vi "Set Channel States and Connections.vi"(8 "error in (no error)":errorcluster, 10 "Routing Channel States":T1, 11 "Channel Ref in":T4 format="%.0x") -> (0 "error out":errorcluster, 3 "Channel Ref out":T4=18446744073709551615 format="%.0x")   [LabVIEW 2017, in "Switch Scripting.lvlib"]
uses:
  Switch Scripting.lvlib
  <vilib>/NI Veristand/Custom Device API/Custom Device Item Ref.ctl
  Channel States.ctl
  Routing State.ctl
  Connection.ctl
  NationalInstruments.VeriStand.SystemDefinitionAPI
  <vilib>/NI VeriStand/Custom Device API/Custom Device API.lvlib
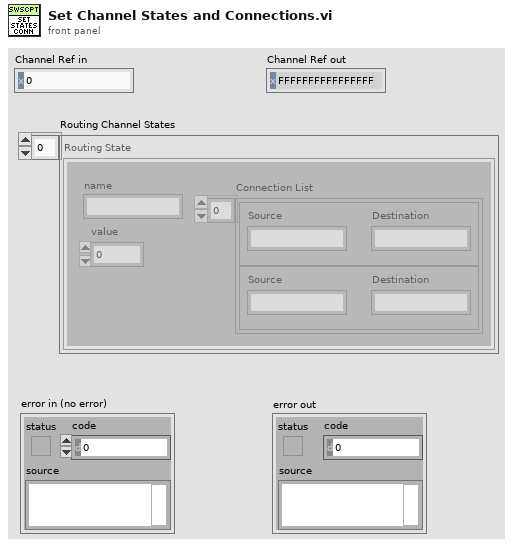
[diagram p1: front panel]
types:
  T1 = typedef "Switch Scripting.lvlib/Channel States.ctl" = T2[]
  T2 = typedef "Switch Scripting.lvlib/Routing State.ctl" = cluster{"name":string, "value":i32, "Connection List":T3[]}
  T3 = typedef "Switch Scripting.lvlib/Connection.ctl" = cluster{"Source":string, "Destination":string}
  T4 = typedef "Custom Device API.lvlib/Custom Device Item Ref.ctl" = u64
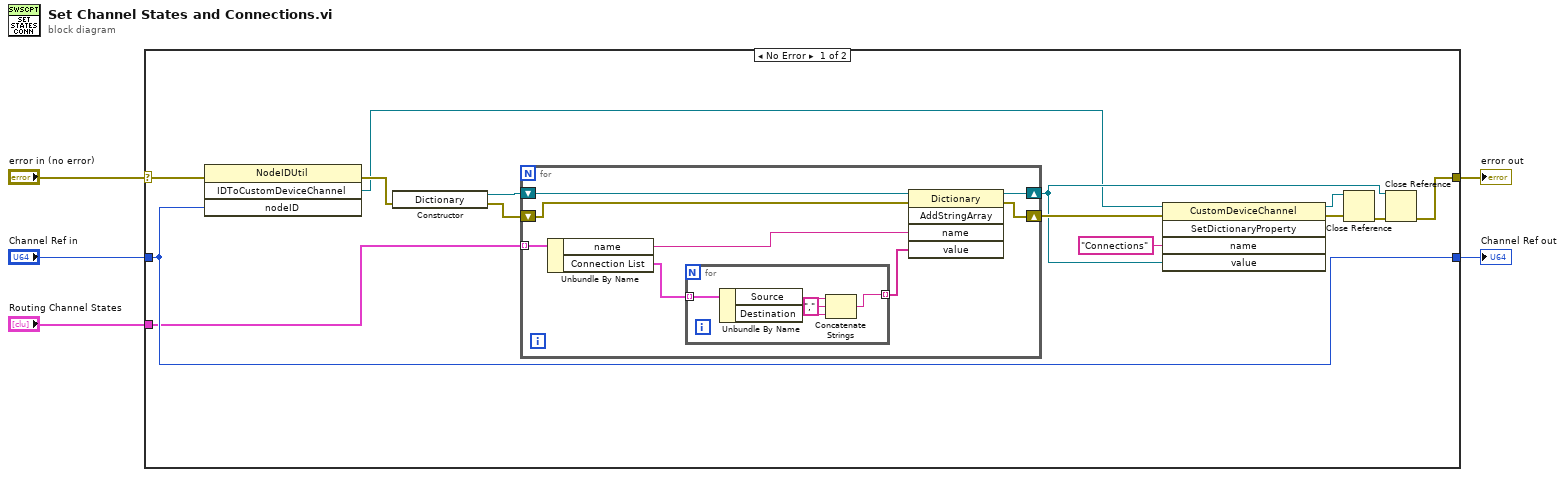
[diagram p0: block diagram]
diagram:
  n1 = case shown="No Error" "error in (no error)" {
    selector: "error in (no error)" -> [w19 w34]
    tunnel: [w18 w34] -> w4
    tunnel: "Channel Ref in" -> [w17 w33]
    tunnel: [w17 w33] -> w2
    tunnel: "Routing Channel States" -> [w16 _]
    frame No Error {
      n2 = invoke class="NodeIDUtil" method="IDToCustomDeviceChannel"(error in=w19, "nodeID"=w17) -> (error out=w15:errorcluster, "IDToCustomDeviceChannel"=w6:refnum<k24>)  [unwired: 2 in, 2 out]
      n3 = constructor class="Dictionary"(error in=w15) -> (reference out=w12:refnum<k24>, error out=w14:errorcluster)  [unwired: 2 in, 1 out]
      n4 = for {
        tunnel: w16 -> [w27] mode=indexing
        shift-right: [w22] -> w11
        shift-left: w14 -> [w23]
        shift-right: [w20] -> w7
        shift-left: w12 -> [w21]
        n5 = Unbundle By Name(w27) -> ("name"=w26:string, "Connection List"=w25:T3[])
        n6 = for {
          tunnel: w25 -> [w32] mode=indexing
          tunnel: [w28] -> w24 mode=indexing
          n7 = Unbundle By Name(w32) -> ("Source"=w31:string, "Destination"=w30:string)
          n8 = Concatenate Strings(w31, "," ("string"), w30) -> (w28:string)
        }
        n9 = invoke class="Dictionary" method="AddStringArray"(reference=w21, error in=w23, "name"=w26, "value"=w24) -> (reference out=w20:refnum<k24>, error out=w22:errorcluster)  [unwired: 1 in, 3 out]
      }
      n10 = invoke class="CustomDeviceChannel" method="SetDictionaryProperty"(reference=w6, error in=w11, "name"="Connections", "value"=w7) -> (reference out=w8:refnum<k24>, error out=w10:errorcluster)  [unwired: 1 in, 3 out]
      n11 = Close Reference(reference=w8, error in (no error)=w10) -> (error out=w9:errorcluster)
      n12 = Close Reference(reference=w7, error in (no error)=w9) -> (error out=w18:errorcluster)
    }
    frame Error {
    }
  }
  "Channel Ref out" <- w2
  "error out" <- w4
